vi "desacade.vi"(0 "Data not diff":dbl[][](array[numeric]), 2 "Capture Saccades":bool, 7 "desacc":T2={"Threshold 1 [Acc]"=0.0, "Threshold 2 [% of TH1]"=0, "tolerance"=2.0, "Search WD "=0.05757575757575758, " always use TH2"=TRUE, "SD for Outliers"=3.0303030303030303, "Max time [ms]"=50.0, "Min time [ms]"=1.0, "Velocity Threshold"=0.05757575757575758} {"Velocity Threshold" scale=50.0..400.0; "SD for Outliers" scale=0.0..5.0; "Search WD" scale=0.0..0.3; "tolerance" scale=0.0..100.0; "Threshold 2 [% of TH1]" scale=0.0..100.0; "Threshold 1 [Acc]" scale=1.0..40000.0}, 9 "Impulse Direction +ve?":bool, 11 "Sample Rate":dbl=500.0 format="%.2f", 12 "Impulse Positions":T1(array[cluster])=[{"Start"=-31, "End"=518, "Impulse Plane"=enum."Other", "Impulse Direction +ve?"=TRUE, "Time offset"=0, "Amplitude offset"=0.0}, {"Start"=369, "End"=913, "Impulse Plane"=enum."Other", "Impulse Direction +ve?"=TRUE, "Time offset"=0, "Amplitude offset"=0.0}, {"Start"=570, "End"=1018, "Impulse Plane"=enum."Other", "Impulse Direction +ve?"=FALSE, "Time offset"=0, "Amplitude offset"=0.0}, {"Start"=770, "End"=1311, "Impulse Plane"=enum."Other", "Impulse Direction +ve?"=TRUE, "Time offset"=0, "Amplitude offset"=0.0}, {"Start"=969, "End"=1417, "Impulse Plane"=enum."Other", "Impulse Direction +ve?"=FALSE, "Time offset"=0, "Amplitude offset"=0.0}, {"Start"=1170, "End"=1708, "Impulse Plane"=enum."Other", "Impulse Direction +ve?"=TRUE, "Time offset"=0, "Amplitude offset"=0.0}, {"Start"=1371, "End"=1819, "Impulse Plane"=enum."Other", "Impulse Direction +ve?"=FALSE, "Time offset"=0, "Amplitude offset"=0.0}, {"Start"=1570, "End"=2104, "Impulse Plane"=enum."Other", "Impulse Direction +ve?"=TRUE, "Time offset"=0, "Amplitude offset"=0.0}, {"Start"=1770, "End"=2218, "Impulse Plane"=enum."Other", "Impulse Direction +ve?"=FALSE, "Time offset"=0, "Amplitude offset"=0.0}, {"Start"=1971, "End"=2508, "Impulse Plane"=enum."Other", "Impulse Direction +ve?"=TRUE, "Time offset"=0, "Amplitude offset"=0.0}, {"Start"=2171, "End"=2619, "Impulse Plane"=enum."Other", "Impulse Direction +ve?"=FALSE, "Time offset"=0, "Amplitude offset"=0.0}, {"Start"=2370, "End"=2917, "Impulse Plane"=enum."Other", "Impulse Direction +ve?"=TRUE, "Time offset"=0, "Amplitude offset"=0.0}, {"Start"=2571, "End"=3019, "Impulse Plane"=enum."Other", "Impulse Direction +ve?"=FALSE, "Time offset"=0, "Amplitude offset"=0.0}, {"Start"=2771, "End"=3308, "Impulse Plane"=enum."Other", "Impulse Direction +ve?"=TRUE, "Time offset"=0, "Amplitude offset"=0.0}, {"Start"=2970, "End"=3418, "Impulse Plane"=enum."Other", "Impulse Direction +ve?"=FALSE, "Time offset"=0, "Amplitude offset"=0.0}, {"Start"=3172, "End"=3715, "Impulse Plane"=enum."Other", "Impulse Direction +ve?"=TRUE, "Time offset"=0, "Amplitude offset"=0.0}, {"Start"=3372, "End"=3820, "Impulse Plane"=enum."Other", "Impulse Direction +ve?"=FALSE, "Time offset"=0, "Amplitude offset"=0.0}, {"Start"=3572, "End"=4107, "Impulse Plane"=enum."Other", "Impulse Direction +ve?"=TRUE, "Time offset"=0, "Amplitude offset"=0.0}, {"Start"=3772, "End"=4220, "Impulse Plane"=enum."Other", "Impulse Direction +ve?"=FALSE, "Time offset"=0, "Amplitude offset"=0.0}, {"Start"=3972, "End"=4512, "Impulse Plane"=enum."Other", "Impulse Direction +ve?"=TRUE, "Time offset"=0, "Amplitude offset"=0.0}, {"Start"=4172, "End"=4620, "Impulse Plane"=enum."Other", "Impulse Direction +ve?"=FALSE, "Time offset"=0, "Amplitude offset"=0.0}, {"Start"=4373, "End"=4920, "Impulse Plane"=enum."Other", "Impulse Direction +ve?"=TRUE, "Time offset"=0, "Amplitude offset"=0.0}, {"Start"=4572, "End"=5020, "Impulse Plane"=enum."Other", "Impulse Direction +ve?"=FALSE, "Time offset"=0, "Amplitude offset"=0.0}, {"Start"=4773, "End"=5315, "Impulse Plane"=enum."Other", "Impulse Direction +ve?"=TRUE, "Time offset"=0, "Amplitude offset"=0.0}, {"Start"=4973, "End"=5421, "Impulse Plane"=enum."Other", "Impulse Direction +ve?"=FALSE, "Time offset"=0, "Amplitude offset"=0.0}, {"Start"=5173, "End"=5716, "Impulse Plane"=enum."Other", "Impulse Direction +ve?"=TRUE, "Time offset"=0, "Amplitude offset"=0.0}, {"Start"=5373, "End"=5821, "Impulse Plane"=enum."Other", "Impulse Direction +ve?"=FALSE, "Time offset"=0, "Amplitude offset"=0.0}, {"Start"=5573, "End"=6110, "Impulse Plane"=enum."Other", "Impulse Direction +ve?"=TRUE, "Time offset"=0, "Amplitude offset"=0.0}, {"Start"=5773, "End"=6221, "Impulse Plane"=enum."Other", "Impulse Direction +ve?"=FALSE, "Time offset"=0, "Amplitude offset"=0.0}, {"Start"=5972, "End"=6515, "Impulse Plane"=enum."Other", "Impulse Direction +ve?"=TRUE, "Time offset"=0, "Amplitude offset"=0.0}, {"Start"=6174, "End"=6622, "Impulse Plane"=enum."Other", "Impulse Direction +ve?"=FALSE, "Time offset"=0, "Amplitude offset"=0.0}, {"Start"=6373, "End"=6913, "Impulse Plane"=enum."Other", "Impulse Direction +ve?"=TRUE, "Time offset"=0, "Amplitude offset"=0.0}, {"Start"=6574, "End"=7022, "Impulse Plane"=enum."Other", "Impulse Direction +ve?"=FALSE, "Time offset"=0, "Amplitude offset"=0.0}, {"Start"=6774, "End"=7314, "Impulse Plane"=enum."Other", "Impulse Direction +ve?"=TRUE, "Time offset"=0, "Amplitude offset"=0.0}, {"Start"=6974, "End"=7422, "Impulse Plane"=enum."Other", "Impulse Direction +ve?"=FALSE, "Time offset"=0, "Amplitude offset"=0.0}, {"Start"=7175, "End"=7712, "Impulse Plane"=enum."Other", "Impulse Direction +ve?"=TRUE, "Time offset"=0, "Amplitude offset"=0.0}, {"Start"=7374, "End"=7822, "Impulse Plane"=enum."Other", "Impulse Direction +ve?"=FALSE, "Time offset"=0, "Amplitude offset"=0.0}, {"Start"=7574, "End"=8111, "Impulse Plane"=enum."Other", "Impulse Direction +ve?"=TRUE, "Time offset"=0, "Amplitude offset"=0.0}, {"Start"=7774, "End"=8222, "Impulse Plane"=enum."Other", "Impulse Direction +ve?"=FALSE, "Time offset"=0, "Amplitude offset"=0.0}, {"Start"=7974, "End"=8518, "Impulse Plane"=enum."Other", "Impulse Direction +ve?"=TRUE, "Time offset"=0, "Amplitude offset"=0.0}, {"Start"=8175, "End"=8623, "Impulse Plane"=enum."Other", "Impulse Direction +ve?"=FALSE, "Time offset"=0, "Amplitude offset"=0.0}, {"Start"=8375, "End"=8920, "Impulse Plane"=enum."Other", "Impulse Direction +ve?"=TRUE, "Time offset"=0, "Amplitude offset"=0.0}, {"Start"=8575, "End"=9023, "Impulse Plane"=enum."Other", "Impulse Direction +ve?"=FALSE, "Time offset"=0, "Amplitude offset"=0.0}, {"Start"=8776, "End"=9315, "Impulse Plane"=enum."Other", "Impulse Direction +ve?"=TRUE, "Time offset"=0, "Amplitude offset"=0.0}, {"Start"=8975, "End"=9423, "Impulse Plane"=enum."Other", "Impulse Direction +ve?"=FALSE, "Time offset"=0, "Amplitude offset"=0.0}, {"Start"=9176, "End"=9715, "Impulse Plane"=enum."Other", "Impulse Direction +ve?"=TRUE, "Time offset"=0, "Amplitude offset"=0.0}, {"Start"=9375, "End"=9823, "Impulse Plane"=enum."Other", "Impulse Direction +ve?"=FALSE, "Time offset"=0, "Amplitude offset"=0.0}, {"Start"=9575, "End"=10110, "Impulse Plane"=enum."Other", "Impulse Direction +ve?"=TRUE, "Time offset"=0, "Amplitude offset"=0.0}], 13 "Display Saccades":bool) -> (4 "Desaccaded":dbl[][](graph), 6 "Mean":dbl[](graph), 8 "STD":dbl[](array[numeric]) format="%.2f", 10 "Mean and STD":dbl[][](array[numeric]) format="%.2f", 14 "Impulse Positions 2":T1(array[cluster]), 15 "Mean (-inf)":dbl[](array[numeric]) format="%.2f")   [LabVIEW 2016]
uses:
  <vilib>/Analysis/3filter.llb/Savitzky-Golay Filter (DBL).vi
  <vilib>/Analysis/NI_AALPro.lvlib
  <vilib>/Analysis/NI_AALBase.lvlib
  stats/stats.lvlib
  nan operations/nan operations.lvlib
panel:
  out "Desaccaded 4":dbl[](graph)
  out "Desaccaded 3":dbl[][](graph)
  out "Desaccaded 2":dbl[](graph)
  out "Data Diff & Quadr - Unsmoothed":dbl[][](graph)
  out "Data DIff & Quadr - Smoothed":dbl[][](graph)
  out "Data not differentiated":dbl[][](graph)
  # "Data Input"
  # "Mean and Standard deviation"
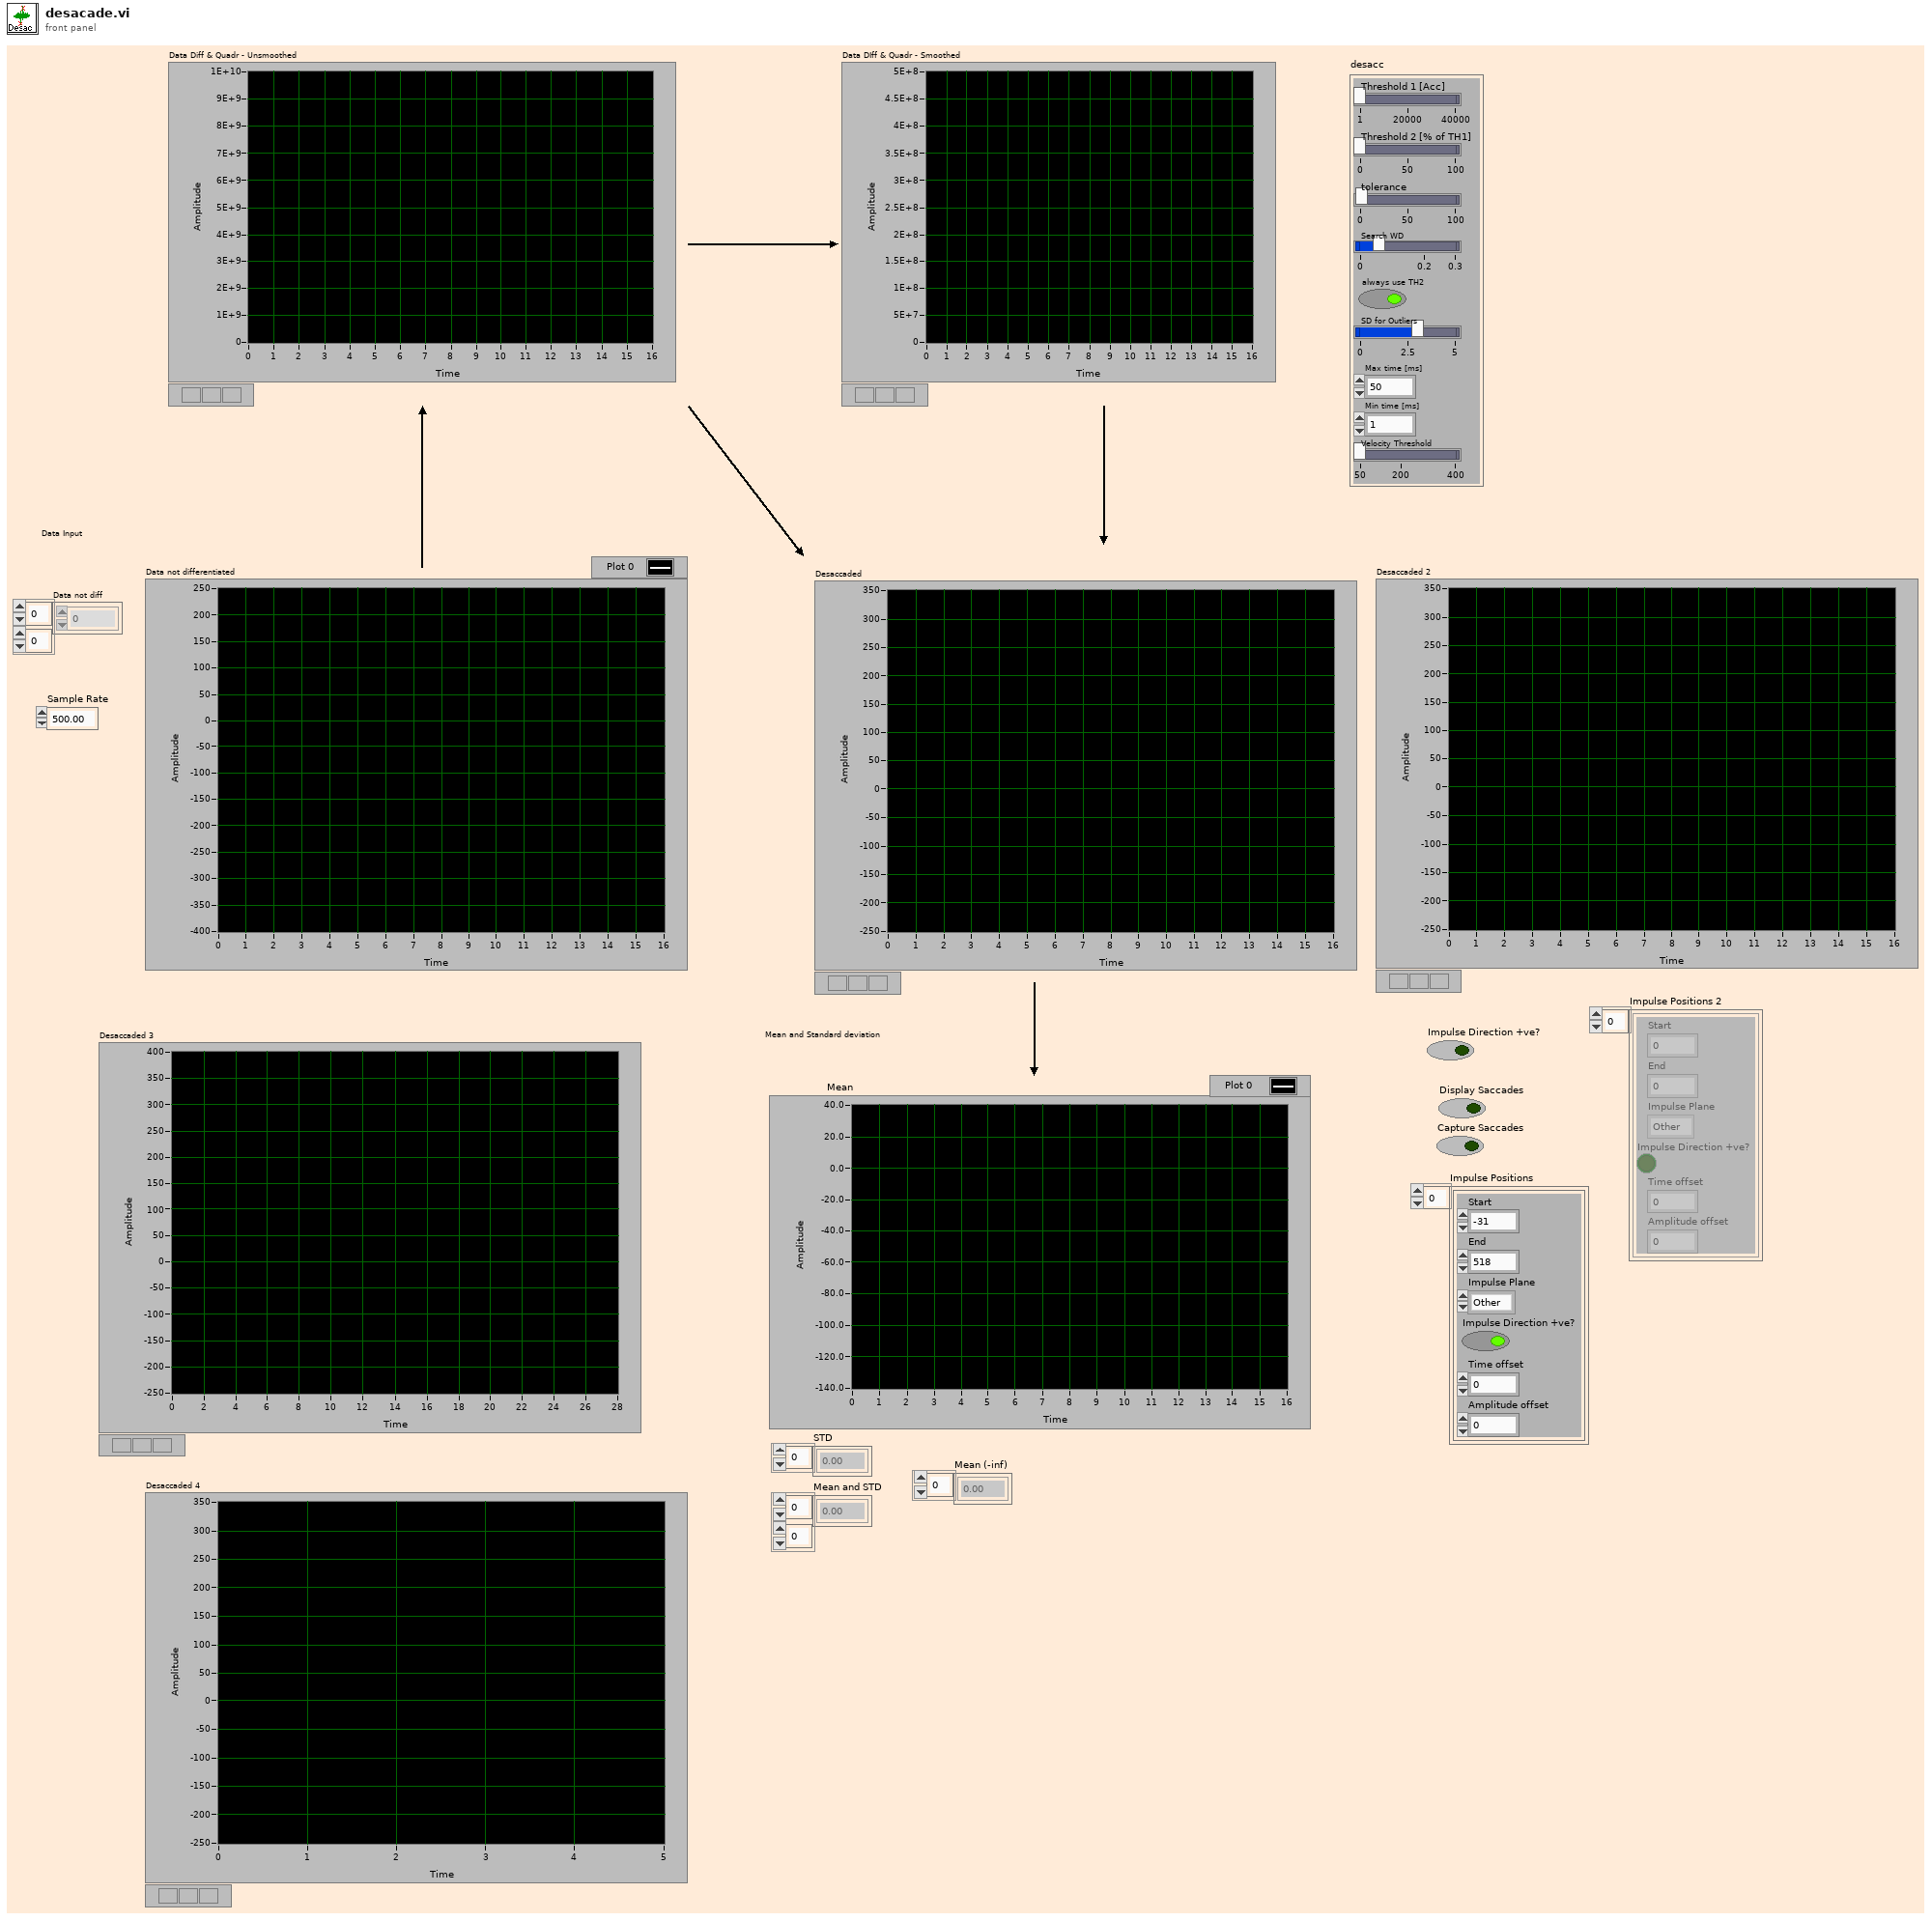
[diagram p1: front panel]
types:
  T1 = cluster{"Start":i32, "End":i32, "Impulse Plane":enum16{"Other", "Yaw", "Pitch", "Roll", "LARP", "RALP"}, "Impulse Direction +ve?":bool, "Time offset":i32, "Amplitude offset":dbl}[]
  T2 = cluster{"Threshold 1 [Acc]":dbl, "Threshold 2 [% of TH1]":i32, "tolerance":dbl, "Search WD ":dbl, " always use TH2":bool, "SD for Outliers":dbl, "Max time [ms]":dbl, "Min time [ms]":dbl, "Velocity Threshold":dbl}
  T3 = cluster{"Start":i32, "End":i32, "Impulse Plane":enum16{"Other", "Yaw", "Pitch", "Roll", "LARP", "RALP"}, "Impulse Direction +ve?":bool, "Time offset":i32, "Amplitude offset":dbl}
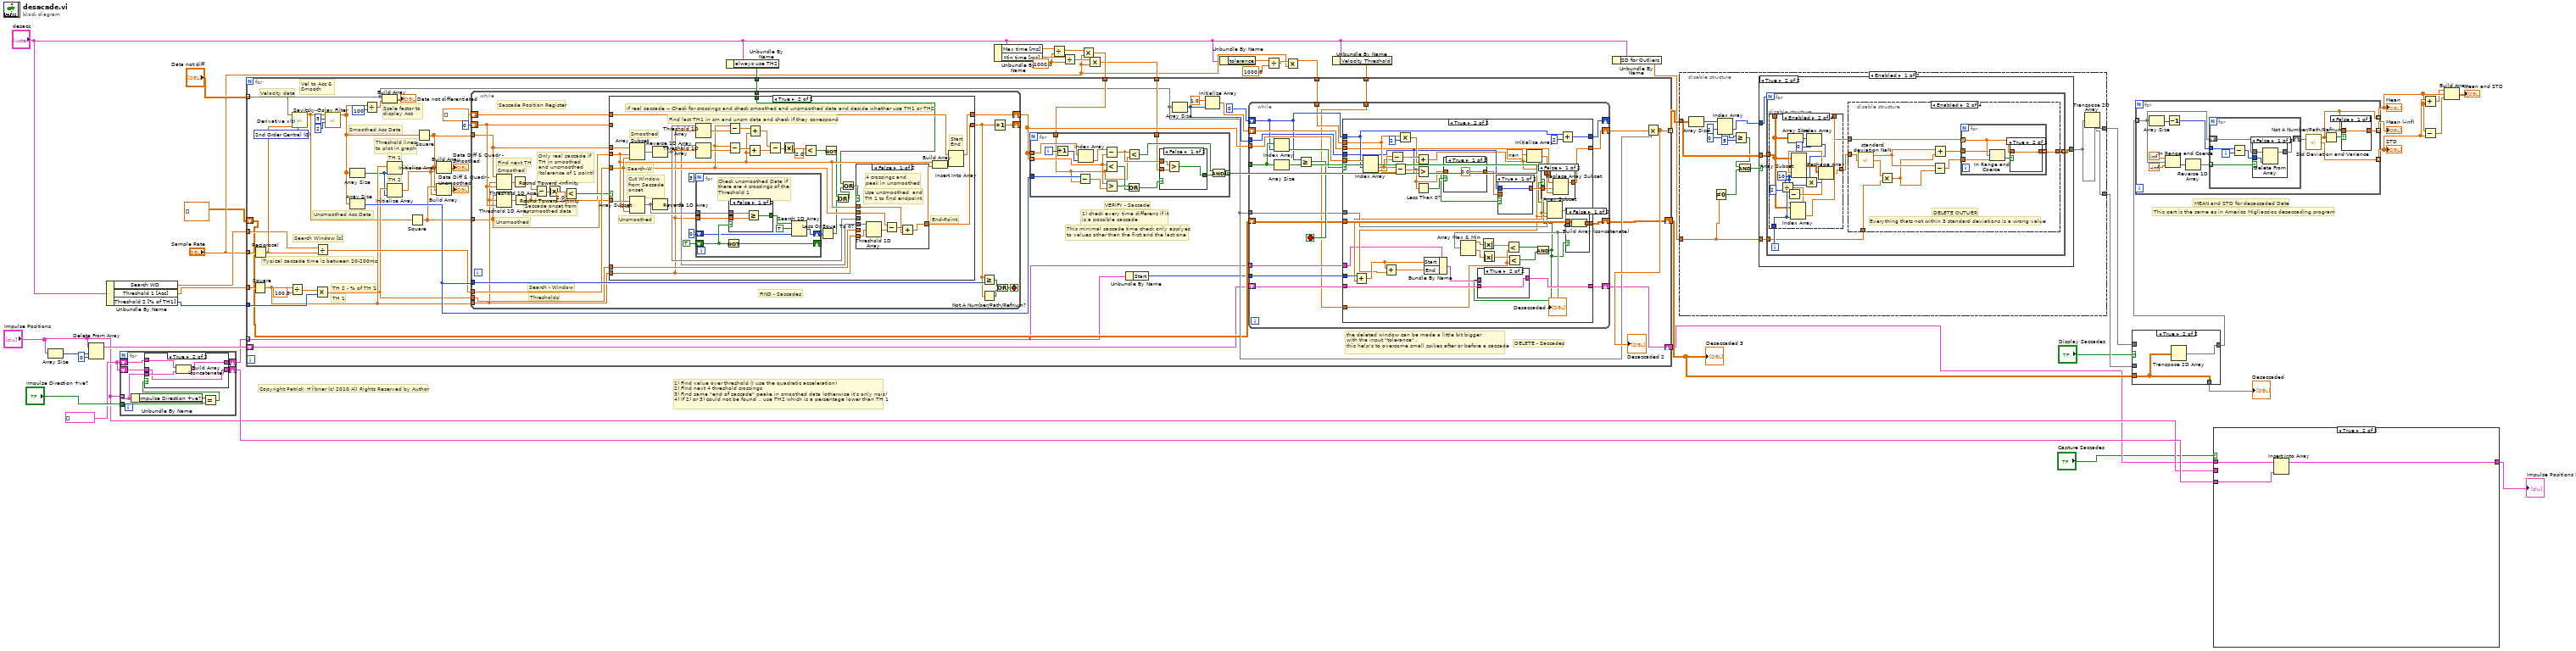
[diagram p0: block diagram]
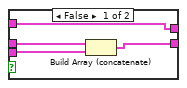
[diagram p3: hidden frame]
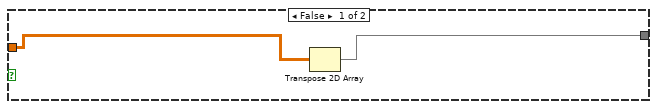
[diagram p5: hidden frame]
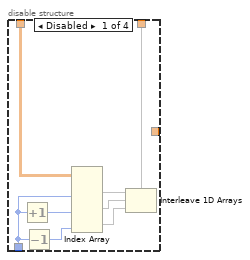
[diagram p6: hidden frame]
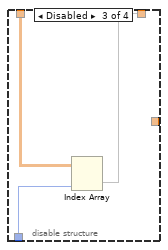
[diagram p7: hidden frame]
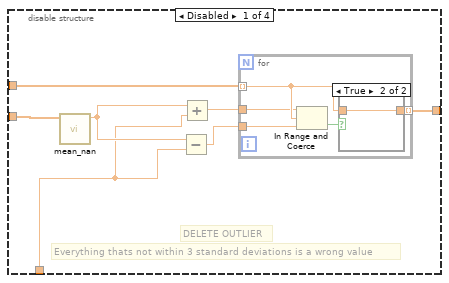
[diagram p9: hidden frame]
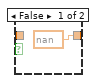
[diagram p10: hidden frame]
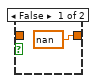
[diagram p11: hidden frame]
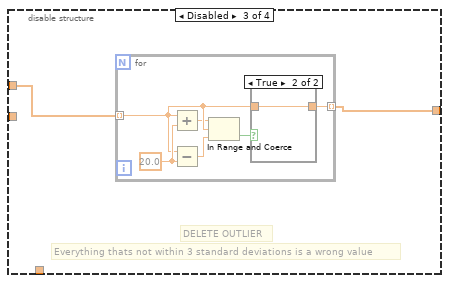
[diagram p12: hidden frame]
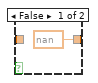
[diagram p13: hidden frame]
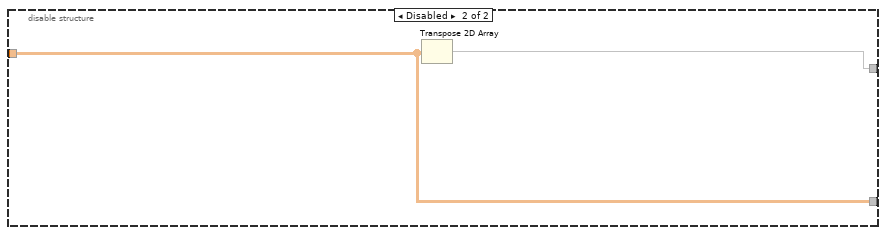
[diagram p15: hidden frame]
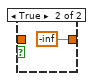
[diagram p17: hidden frame]
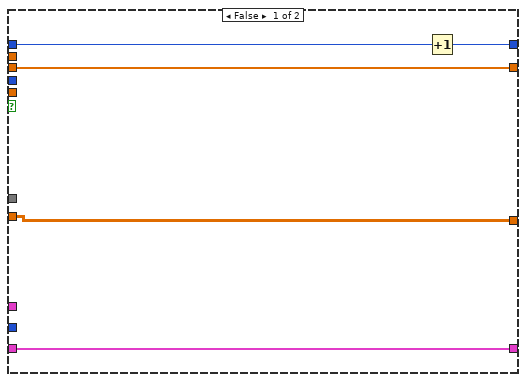
[diagram p18: hidden frame]
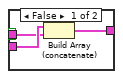
[diagram p20: hidden frame]
diagram:
  w8 = T1 []
  w30 = 1000.0 ("y")
  # "This part is the same as in Americo Migliaccios desaccading program"
  # "MEAN and STD for desaccaded Data"
  # "1) Find value over threshold (I use the quadratic acceleration)\n2) Find next 4 threshold crossings\n3) Find same \"end of saccade\" peake in smoothed data (otherwise it's only nois)\n4) If 2) or 3) could not be found .. use TH2 which is a persentage lower than TH 1"
  # "Copyright Patrick  HŸbner (c) 2010 All Rights Reserved by Author"
  n1 = Array Size(array="Impulse Positions") -> (size(s)=w11:i32)
  n2 = Delete From Array(array="Impulse Positions", length=w11, index=0) -> (array with subset deleted=w13:T1)  [unwired: 1 out]
  n3 = Unbundle By Name("desacc") -> ("Search WD"=w37:dbl, "Threshold 1 [Acc]"=w36:dbl, "Threshold 2 [% of TH1]"=w35:i32)
  n4 = for {
    tunnel: "Impulse Positions" -> [w48] mode=indexing
    tunnel: "Impulse Direction +ve?" -> [w52]
    shift-right: [w49] -> w9
    shift-left: w8 -> [w50]
    shift-right: [w46] -> w7
    shift-left: w8 -> [w47]
    n5 = Unbundle By Name(w48) -> ("Impulse Direction +ve?"=w53:bool)
    n6 = Equal?(x=w53, y=w52) -> (x = y?=w51:bool)
    n7 = case shown="True" w51 {
      tunnel: w48 -> [w56 w61]
      tunnel: w50 -> [w57 w60]
      tunnel: [w57 w59] -> w49
      tunnel: w47 -> [w55 w58]
      tunnel: [w54 w58] -> w46
      frame False {
        n8 = Build Array (concatenate)(w55, w56) -> (w54:T1)
      }
      frame True {
        n9 = Build Array (concatenate)(w60, w61) -> (w59:T1)
      }
    }
  }
  n10 = Unbundle By Name("desacc") -> ("always use TH2"=w34:bool)
  n11 = Unbundle By Name("desacc") -> ("Max time [ms]"=w32:dbl, "Min time [ms]"=w31:dbl)
  n12 = Divide(x=w32, y=w30) -> (x/y=w29:dbl)
  n13 = Divide(x=w31, y=w30) -> (x/y=w28:dbl)
  n14 = Multiply(x=w29, y="Sample Rate") -> (x*y=w27:dbl)
  n15 = Multiply(x=w28, y="Sample Rate") -> (x*y=w26:dbl)
  n16 = Unbundle By Name("desacc") -> ("tolerance"=w25:dbl)
  n17 = Divide(x=w25, y=1000.0) -> (x/y=w22:dbl)
  n18 = Multiply(x=w22, y="Sample Rate") -> (x*y=w23:dbl)
  n19 = Unbundle By Name("desacc") -> ("Velocity Threshold"=w1:dbl)
  n20 = for {
    tunnel: "Sample Rate" -> [w109]
    tunnel: w36 -> [w106]
    tunnel: "Data not diff" -> [w70] mode=indexing
    tunnel: [w76] -> w38 mode=indexing
    tunnel: w35 -> [w92]
    tunnel: w37 -> [w75]
    tunnel: w34 -> [w74]
    tunnel: w27 -> [w73]
    tunnel: w23 -> [w72]
    tunnel: w26 -> [w71]
    shift-right: [w69] -> w17
    shift-left: dbl[][] [] -> [w68]
    tunnel: w9 -> [w67] mode=indexing
    shift-right: [w64] -> w5
    shift-left: w13 -> [w65]
    tunnel: w1 -> [w63]
    w108 = u16 0 items=["2nd Order Central", "4th Order Central", "Forward", "Backward"] ("method")
    # "DELETE - Saccades"
    # "Scale factor to \ndisplay Acc"
    # "This minimal saccade time check only applyes \nto values other than the first and the last one"
    # "VERIFY - Saccade"
    # "Threshold lines \nto plot in graph"
    # "TH 2"
    # "TH 1"
    # "Vel to Acc &\nSmooth"
    # "Unsmoothed Acc Data"
    # "Smoothed Acc Data"
    # "Velocity data"
    # "Typical saccade time is between 20-200ms"
    # "Search Window [s]"
    # "TH 1"
    # "TH 2 - % of TH 1"
    # "the deleted window can be made a little bit bigger \nwith the input \"tolerance\" . \nthis help's to overcome small spikes after or before a saccade"
    # "1) check every time differenz if it \nis a possible saccade"
    n21 = Square(x=w106) -> (x^2=w88:dbl)
    n22 = Reciprocal(x=w109) -> (1/x=w79:dbl)
    n23 = Divide(x=w88, y=100.0) -> (x/y=w93:dbl)
    n24 = call <vilib>:"Derivative x(t).vi"("method"=w108, "dt"=w79, "X"=w70) -> ("dX/dt"=w62:dbl[])  [unwired: 7 in, 1 out]
    n25 = Multiply(x=w93, y=w92) -> (x*y=w87:dbl)
    n26 = Divide(x=w75, y=w79) -> (x/y=w89:dbl)
    n27 = call-poly <vilib>:"Savitzky-Golay Filter.vi"("polynomial order"=2, "side points"=5, "X"=w62) -> ("Filtered X"=w78:dbl[])  [unwired: 7 in, 1 out]
    n28 = Array Size(array=w78) -> (size(s)=w86:i32)
    n29 = Array Size(array=w78) -> (size(s)=w99:i32)
    n30 = Divide(x=w78, y=100 ("Numeric")) -> (x/y=w96:dbl[])
    n31 = Build Array(w70, w96) -> (→"Data not differentiated":dbl[][])
    n32 = Initialize Array(w88, w86) -> (w81:dbl[])
    n33 = Initialize Array(w87, w86) -> (w80:dbl[])
    n34 = Square(x=w62) -> (x^2=w83:dbl[])
    n35 = Square(x=w78) -> (x^2=w82:dbl[])
    n36 = Build Array(w82, w81, w80) -> (→"Data DIff & Quadr - Smoothed":dbl[][])
    n37 = Build Array(w83, w81, w80) -> (→"Data Diff & Quadr - Unsmoothed":dbl[][])
    n38 = while {
      tunnel: w82 -> [w217]
      shift-right: [w231] -> _
      shift-left: 0 -> [w220]
      shift-right: [w232] -> w101
      shift-left: dbl[] [] ("Filtered X") -> [w230]
      tunnel: w99 -> [w225]
      tunnel: w83 -> [w216]
      tunnel: w89 -> [w222]
      tunnel: w87 -> [w218]
      tunnel: w88 -> [w219]
      tunnel: w74 -> [w211]
      stop <- w224 stop-if-true
      # "FIND - Saccades"
      # "Saccade Position Register"
      # "Only real saccade if\nTH in smoothed\nand unsmoothed \n(tolerance of 1 point)"
      # "Unsmoothed"
      # "Smoothed"
      # "Saccade onset from\nunsmoothed data"
      # "Search - Window"
      # "Thresholds"
      # "Find next TH"
      n39 = Threshold 1D Array(1:w220, 2:w219, 3:w217) -> (0:w233:dbl)
      n40 = Threshold 1D Array(1:w220, 2:w219, 3:w216) -> (0:w229:dbl)
      n41 = Round Toward -Infinity(1:w233) -> (0:w215:dbl)
      n42 = Round Toward -Infinity(1:w229) -> (0:w214:dbl)
      n43 = Subtract(x=w215, y=w214) -> (x-y=w228:dbl)
      n44 = Absolute Value(x=w228) -> (abs(x)=w227:dbl)
      n45 = Less?(x=w227, y=2.0) -> (x < y?=w221:bool)
      n46 = case shown="True" w221 {
        tunnel: [w234 w268] -> w232
        tunnel: w230 -> [w234 w267]
        tunnel: w216 -> [_ w259]
        tunnel: w217 -> [_ w258]
        tunnel: w218 -> [_ w247]
        tunnel: [w235 w246] -> w223
        tunnel: w222 -> [_ w245]
        tunnel: w214 -> [_ w244]
        tunnel: w219 -> [_ w242]
        tunnel: w220 -> [w235 _]
        tunnel: w211 -> [_ w236]
        frame False {
          # "If no real saccade -- Do nothing"
        }
        frame True {
          # "End-Point"
          # "If real saccade -- Check for crossings and check smoothed and unsmoothed data and deside whether use TH1 or TH2"
          # "Find last TH1 in sm and unsm data and check if they correspond"
          # "Smoothed"
          # "Unsmoothed"
          # "Cut Window \nfrom Saccade\nonset"
          # "Search-W"
          # "Start\nEnd"
          n47 = Array Subset(array=w258, index=w244, length=w245) -> (w257:dbl[])
          n48 = Array Subset(array=w259, index=w244, length=w245) -> (w263:dbl[])
          n49 = Reverse 1D Array(array=w257) -> (reversed array=w248:dbl[])
          n50 = Reverse 1D Array(array=w263) -> (reversed array=w243:dbl[])
          n51 = Threshold 1D Array(2:w242, 3:w248) -> (0:w249:dbl)  [unwired: 1 in]
          n52 = Threshold 1D Array(2:w242, 3:w243) -> (0:w256:dbl)  [unwired: 1 in]
          n53 = for {
            N: 3 -> [_]
            tunnel: w263 -> [w290]
            shift-right: [w285] -> _
            shift-left: TRUE -> [w284]
            tunnel: w242 -> [w289]
            shift-right: [w286] -> w260
            shift-left: 0 ("index of element") -> [w283]
            # "Check unsmoothed Data if \nthere are 4 crossings of the \nThreshold 1"
            n54 = Not(x=w284) -> (.not. x?=w285:bool)
            n55 = case shown="False" w284 {
              tunnel: w290 -> [w293 w296]
              tunnel: w289 -> [w292 w295]
              tunnel: [w291 w294] -> w288
              frame False {
                n56 = Greater Or Equal?(x=w293, y=w292) -> (x >= y?=w291:bool[])
              }
              frame True {
                n57 = Less?(x=w296, y=w295) -> (x < y?=w294:bool[])
              }
            }
            n58 = Search 1D Array(1D array=w288, element=TRUE, start index (0)=w283) -> (index of element=w286:i32)
          }
          n59 = Subtract(x=w245, y=w249) -> (x-y=w255:dbl)
          n60 = Subtract(x=w245, y=w256) -> (x-y=w265:dbl)
          n61 = Add(x=w265, y=w244) -> (x+y=w250:dbl)
          n62 = Add(x=w255, y=w244) -> (x+y=w251:dbl)
          n63 = Subtract(x=w251, y=w250) -> (x-y=w254:dbl)
          n64 = Absolute Value(x=w254) -> (abs(x)=w253:dbl)
          n65 = Less?(x=w253, y=2.0) -> (x < y?=w241:bool)
          n66 = Less Or Equal To 0?(x=w260) -> (x <= 0?=w240:bool)
          n67 = Not(x=w241) -> (.not. x?=w239:bool)
          n68 = Or(x=w239, y=w240) -> (x .or. y?=w238:bool)
          n69 = Or(x=w236, y=w238) -> (x .or. y?=w237:bool)
          n70 = case shown="False" w237 {
            tunnel: w248 -> [_ w280]
            tunnel: w247 -> [_ w279]
            tunnel: [w273 w278] -> w246
            tunnel: w245 -> [w272 w277]
            tunnel: w244 -> [w271 w276]
            tunnel: w243 -> [w270 _]
            tunnel: w242 -> [w269 _]
            frame False {
              # "Use unsmoothed  and\nTH 1 to find endpoint"
              # "4 crossings and\npeak in unsmoothed"
              n71 = Threshold 1D Array(2:w269, 3:w270) -> (0:w274:dbl)  [unwired: 1 in]
              n72 = Subtract(x=w272, y=w274) -> (x-y=w275:dbl)
              n73 = Add(x=w275, y=w271) -> (x+y=w273:dbl)
            }
            frame True {
              # "Use smoothed data and\nTH 2 to find endpoint"
              # "not 4 crossings or \nno peak in unsmoothed"
              n74 = Threshold 1D Array(2:w279, 3:w280) -> (0:w281:dbl)  [unwired: 1 in]
              n75 = Subtract(x=w277, y=w281) -> (x-y=w282:dbl)
              n76 = Add(x=w282, y=w276) -> (x+y=w278:dbl)
            }
          }
          n77 = Build Array(w244, w246) -> (w266:dbl[])
          n78 = Insert Into Array(array=w267, new element=w266) -> (w268:dbl[])  [unwired: 1 in]
        }
      }
      n79 = Greater Or Equal?(x=w223, y=w225) -> (x >= y?=w213:bool)
      n80 = Not A Number/Path/Refnum?(number/path/refnum=w223) -> (NaN/Path/Refnum?=w212:bool)
      n81 = Increment(x=w223) -> (x+1=w231:dbl)
      n82 = Or(x=w213, y=w212) -> (x .or. y?=w224:bool)
    }
    n83 = for {
      tunnel: w101 -> [w195] mode=indexing
      tunnel: w101 -> [w206]
      tunnel: [w201] -> w104 mode=indexing
      tunnel: w99 -> [w193]
      tunnel: w73 -> [w192]
      tunnel: w71 -> [w191]
      i -> [w199]
      n84 = Increment(x=w199) -> (x+1=w205:i32)
      n85 = Subtract(x=w193, y=w192) -> (x-y=w194:dbl)
      n86 = Index Array(array=w206, index=w205) -> (element=w204:dbl)
      n87 = Subtract(x=w204, y=w195) -> (x-y=w200:dbl)
      n88 = Less?(x=w195, y=w192) -> (x < y?=w196:bool)
      n89 = Greater?(x=w195, y=w194) -> (0:w198:bool)
      n90 = Less?(x=w200, y=w192) -> (x < y?=w203:bool)
      n91 = Or(x=w198, y=w196) -> (x .or. y?=w197:bool)
      n92 = case shown="False" w197 {
        tunnel: w191 -> [w209 _]
        tunnel: [w208 TRUE] -> w202
        tunnel: w200 -> [w207 _]
        frame False {
          n93 = Greater?(x=w207, y=w209) -> (0:w208:bool)
        }
        frame True {
        }
      }
      n94 = And(x=w203, y=w202) -> (x .and. y?=w201:bool)
    }
    n95 = Unbundle By Name(w67) -> ("Start"=w66:i32)
    n96 = Array Size(array=w70) -> (size(s)=w98:i32)
    n97 = Initialize Array(1.0 ("element"), w98) -> (w102:dbl[])
    n98 = while {
      tunnel: w101 -> [w127]
      shift-right: [w125] -> w77
      shift-left: w102 -> [w126]
      shift-right: [w123] -> _
      shift-left: 0 -> [w120]
      tunnel: w104 -> [w124]
      tunnel: w98 -> [w119]
      tunnel: w72 -> [w118]
      shift-right: [w117] -> w69
      shift-left: w68 -> [w116]
      tunnel: w70 -> [w115]
      tunnel: w67 -> [w114]
      tunnel: w66 -> [w113]
      shift-right: [w111] -> w64
      shift-left: w65 -> [w112]
      tunnel: w63 -> [w110]
      stop <- w122 stop-if-true
      n99 = Index Array(array=w124, index=w120) -> (element=w128:bool)
      n100 = Array Size(array=w124) -> (size(s)=w121:i32)
      n101 = Greater Or Equal?(x=w120, y=w121) -> (x >= y?=w122:bool)
      n102 = case shown="True" w128 {
        tunnel: w127 -> [_ w173]
        tunnel: w126 -> [w133 w152]
        tunnel: [w133 w168] -> w125
        tunnel: w120 -> [w132 w166]
        tunnel: [w131 w167] -> w123
        tunnel: w118 -> [_ w161]
        tunnel: w119 -> [_ w156]
        tunnel: [w130 w155] -> w117
        tunnel: w116 -> [w130 w154]
        tunnel: w115 -> [_ w153]
        tunnel: w114 -> [_ w146]
        tunnel: w113 -> [_ w151]
        tunnel: w112 -> [w129 w145]
        tunnel: [w129 w143] -> w111
        tunnel: w110 -> [_ w134]
        frame False {
          n103 = Increment(x=w132) -> (x+1=w131:i32)
        }
        frame True {
          n104 = Index Array(array=w173, index #1=w166) -> (element #1=w162:dbl, element #2=w172:dbl)  [unwired: 1 in]
          n105 = Subtract(x=w172, y=w162) -> (x-y=w170:dbl)
          n106 = Subtract(x=w162, y=w161) -> (x-y=w159:dbl)
          n107 = Multiply(x=w161, y=2) -> (x*y=w163:dbl)
          n108 = Add(x=w170, y=w163) -> (x+y=w148:dbl)
          n109 = Greater?(x=w159, y=w156) -> (0:w158:bool)
          n110 = Less Than 0?(x=w159) -> (x < 0?=w160:bool)
          n111 = case shown="True" w160 {
            tunnel: w159 -> [_ w190]
            tunnel: [0.0 w190] -> w157
            frame True {
            }
            frame False {
            }
          }
          n112 = case shown="True" w158 {
            tunnel: w157 -> [_ w188]
            tunnel: [w187 w188] -> w150
            tunnel: w156 -> [w187 _]
            frame True {
            }
            frame False {
            }
          }
          n113 = Add(x=w151, y=w150) -> (x+y=w149:dbl)
          n114 = Add(x=w149, y=w148) -> (x+y=w147:dbl)
          n115 = Bundle By Name(cluster=w146, "Start"=w149, "End"=w147) -> (w144:T3)
          n116 = Initialize Array(nan, w148) -> (w169:dbl[])
          n117 = Array Subset(array=w153, index=w150, length=w148) -> (w136:dbl[])
          "Desaccaded 4" <- w136
          n118 = Array Max & Min(array=w136) -> (max value=w142:dbl, min value=w141:dbl)  [unwired: 2 out]
          n119 = Absolute Value(x=w142) -> (abs(x)=w140:dbl)
          n120 = Absolute Value(x=w141) -> (abs(x)=w139:dbl)
          n121 = Less?(x=w140, y=w134) -> (x < y?=w138:bool)
          n122 = Less?(x=w139, y=w134) -> (x < y?=w137:bool)
          n123 = And(x=w138, y=w137) -> (x .and. y?=w135:bool)
          n124 = case shown="True" w135 {
            tunnel: w145 -> [w180 w181]
            tunnel: w144 -> [w179 _]
            tunnel: [w178 w181] -> w143
            frame False {
              n125 = Build Array (concatenate)(w180, w179) -> (w178:T1)
            }
            frame True {
            }
          }
          n126 = case shown="False" w135 {
            tunnel: w169 -> [w185 _]
            tunnel: [w184 w186] -> w168
            tunnel: w152 -> [w183 w186]
            tunnel: w150 -> [w182 _]
            frame False {
              n127 = Replace Array Subset(array=w183, new element=w185, index=w182) -> (w184:dbl[])
            }
            frame True {
            }
          }
          n128 = Add(x=w166, y=2) -> (x+y=w167:i32)
          n129 = case shown="False" w135 {
            tunnel: [w176 w177] -> w155
            tunnel: w154 -> [w175 w177]
            tunnel: w136 -> [w174 _]
            frame False {
              n130 = Build Array (concatenate)(w175, w174) -> (w176:dbl[][])
            }
            frame True {
            }
          }
        }
      }
    }
    n131 = Multiply(x=w77, y=w70) -> (x*y=w76:dbl[])
    "Desaccaded 2" <- w76
  }
  "Desaccaded 3" <- w17
  n132 = Unbundle By Name("desacc") -> ("SD for Outliers"=w33:dbl)
  n133 = disable-structure shown="Enabled" {
    disable-tunnel: [w307 w386] -> w16
    disable-tunnel: [w306 w385] -> w19
    disable-tunnel: w38 -> [w305 w385]
    disable-tunnel: w33 -> [w297 _]
    frame Enabled {
      n134 = Array Size(array=w305) -> (size(s)=w309:i32[])
      n135 = Not Equal To 0?(x=w297) -> (x != 0?=w298:bool)
      n136 = Index Array(array=w309, index #1=1 ("index"), index #2=0 ("index")) -> (element #1=w304:i32, element #2=w302:i32)
      n137 = Greater Or Equal?(x=w302, y=5) -> (x >= y?=w299:bool)
      n138 = And(x=w299, y=w298) -> (x .and. y?=w300:bool)
      n139 = case shown="True" w300 {
        tunnel: [w310 w315] -> w307
        tunnel: w305 -> [w311 w314]
        tunnel: w304 -> [_ w313]
        tunnel: w297 -> [_ w312]
        frame False {
          n140 = Transpose 2D Array(2D array=w311) -> (transposed array=w310:dbl[][])
        }
        frame True {
          n141 = for {
            N: w313 -> [_]
            tunnel: w314 -> [w320]
            tunnel: [w321] -> w315 mode=indexing
            tunnel: w312 -> [w317]
            i -> [w318]
            n142 = disable-structure shown="Enabled" {
              disable-tunnel: w320 -> [w328 w334 w344 _]
              disable-tunnel: [w324 w341 w342 _] -> w319
              disable-tunnel: w318 -> [w322 w338 w343 _]
              disable-tunnel: [_ w336 _ _] -> w316
              frame Disabled {
                n143 = Increment(x=w322) -> (x+1=w327:i32)
                n144 = Decrement(x=w322) -> (x-1=w323:i32)
                n145 = Index Array(array=w328, index (col) #1=w322, index (col) #2=w327, index (col) #3=w323) -> (element #1=w324:dbl[], element #2=w326:dbl[], element #3=w325:dbl[])  [unwired: 3 in]
                n146 = Interleave 1D Arrays(w324, w326, w325) -> ()  [unwired: 1 out]
              }
              frame Enabled {
                w332 = 10 ("length")
                n147 = Divide(x=w332, y=2) -> (x/y=w337:dbl)
                n148 = Subtract(x=w338, y=w337) -> (x-y=w340:dbl)
                n149 = Array Size(array=w334) -> (size(s)=w331:i32[])
                n150 = Index Array(array=w334, index (col)=w338) -> (element=w341:dbl[])  [unwired: 1 in]
                n151 = Array Subset(array=w334, index (col)=w340, length (col)=w332) -> (w335:dbl[][])  [unwired: 2 in]
                n152 = Index Array(array=w331, index=0) -> (element=w330:i32)
                n153 = Multiply(x=w330, y=w332) -> (x*y=w329:i32)
                n154 = Reshape Array(w335, w329) -> (w336:dbl[])
              }
              frame Disabled {
                n155 = Index Array(array=w344, index (col)=w343) -> (element=w342:dbl[])  [unwired: 1 in]
              }
              frame Disabled {
              }
            }
            n156 = disable-structure shown="Enabled" {
              disable-tunnel: [w351 w367 w376 _] -> w321
              disable-tunnel: w316 -> [w350 w366 _ _]
              disable-tunnel: w319 -> [w349 w365 w375 _]
              disable-tunnel: w317 -> [w345 w360 _ _]
              frame Disabled {
                # "DELETE OUTLIER"
                # "Everything thats not within 3 standard deviations is a wrong value"
                n157 = call "mean_nan.vi"("Array"=w350) -> ("Mean"=w348:dbl)  [unwired: 10 in]
                n158 = Subtract(x=w348, y=w345) -> (x-y=w347:dbl)
                n159 = Add(x=w348, y=w345) -> (x+y=w346:dbl)
                n160 = for {
                  tunnel: [w355] -> w351 mode=indexing
                  tunnel: w349 -> [w354] mode=indexing
                  tunnel: w347 -> [w353]
                  tunnel: w346 -> [w352]
                  n161 = In Range and Coerce(upper limit=w352, x=w354, lower limit=w353) -> (In Range?=w356:bool)  [unwired: 1 out]
                  n162 = case shown="True" w356 {
                    tunnel: [nan w358] -> w355
                    tunnel: w354 -> [_ w358]
                    frame False {
                    }
                    frame True {
                    }
                  }
                }
              }
              frame Enabled {
                # "DELETE OUTLIER"
                # "Everything thats not within 3 standard deviations is a wrong value"
                n163 = call "standard deviation NaN.vi"("Array"=w366) -> ("standard deviation"=w361:dbl, "mean"=w364:dbl)  [unwired: 2 in, 1 out]
                n164 = Multiply(x=w361, y=w360) -> (x*y=w359:dbl)
                n165 = Subtract(x=w364, y=w359) -> (x-y=w363:dbl)
                n166 = Add(x=w364, y=w359) -> (x+y=w362:dbl)
                n167 = for {
                  tunnel: [w371] -> w367 mode=indexing
                  tunnel: w365 -> [w370] mode=indexing
                  tunnel: w363 -> [w369]
                  tunnel: w362 -> [w368]
                  n168 = In Range and Coerce(upper limit=w368, x=w370, lower limit=w369) -> (In Range?=w372:bool)  [unwired: 1 out]
                  n169 = case shown="True" w372 {
                    tunnel: [nan w374] -> w371
                    tunnel: w370 -> [_ w374]
                    frame False {
                    }
                    frame True {
                    }
                  }
                }
              }
              frame Disabled {
                # "DELETE OUTLIER"
                # "Everything thats not within 3 standard deviations is a wrong value"
                n170 = for {
                  tunnel: [w381] -> w376 mode=indexing
                  tunnel: w375 -> [w379] mode=indexing
                  w380 = 20.0 ("y")
                  n171 = Add(x=w379, y=w380) -> (x+y=w377:dbl)
                  n172 = Subtract(x=w379, y=w380) -> (x-y=w378:dbl)
                  n173 = In Range and Coerce(upper limit=w377, x=w379, lower limit=w378) -> (In Range?=w382:bool)  [unwired: 1 out]
                  n174 = case shown="True" w382 {
                    tunnel: [nan w384] -> w381
                    tunnel: w379 -> [_ w384]
                    frame False {
                    }
                    frame True {
                    }
                  }
                }
              }
              frame Disabled {
              }
            }
          }
        }
      }
      n175 = Transpose 2D Array(2D array=w307) -> (transposed array=w306:dbl[][])
    }
    frame Disabled {
      n176 = Transpose 2D Array(2D array=w385) -> (transposed array=w386:dbl[][])
    }
  }
  n177 = case shown="True" "Display Saccades" {
    tunnel: w19 -> [w388 _]
    tunnel: [w388 w389] -> w18
    tunnel: w17 -> [_ w389]
    tunnel: [w387 w390] -> w15
    tunnel: w16 -> [w387 _]
    frame False {
    }
    frame True {
      n178 = Transpose 2D Array(2D array=w389) -> (transposed array=w390:dbl[][])
    }
  }
  "Desaccaded" <- w18
  n179 = for {
    tunnel: w15 -> [w393] mode=indexing
    tunnel: [w399] -> w43 mode=indexing
    tunnel: [w402] -> w44 mode=indexing
    tunnel: [w400] -> w39 mode=indexing
    n180 = Array Size(array=w393) -> (size(s)=w392:i32)
    n181 = In Range and Coerce(upper limit=inf, x=w393, lower limit=-inf) -> (In Range?=w395:bool[])  [unwired: 1 out]
    n182 = Decrement(x=w392) -> (x-1=w391:i32)
    n183 = Reverse 1D Array(array=w395) -> (reversed array=w394:bool[])
    n184 = for {
      tunnel: w394 -> [w408] mode=indexing
      shift-right: [w406] -> w398
      shift-left: w393 -> [w407]
      tunnel: w391 -> [w405]
      i -> [w404]
      n185 = Subtract(x=w405, y=w404) -> (x-y=w403:i32)
      n186 = case shown="False" w408 {
        tunnel: w407 -> [w411 w412]
        tunnel: [w409 w412] -> w406
        tunnel: w403 -> [w410 _]
        frame False {
          n187 = Delete From Array(array=w411, index=w410) -> (array with subset deleted=w409:dbl[])  [unwired: 1 in, 1 out]
        }
        frame True {
        }
      }
    }
    n188 = call "Std Deviation and Variance.vi"("X"=w398) -> ("mean"=w399:dbl, "standard deviation"=w402:dbl)  [unwired: 1 in, 1 out]
    n189 = Not A Number/Path/Refnum?(number/path/refnum=w399) -> (NaN/Path/Refnum?=w401:bool)
    n190 = case shown="False" w401 {
      tunnel: [w413 -inf] -> w400
      tunnel: w399 -> [w413 _]
      frame False {
      }
      frame True {
      }
    }
  }
  "Mean" <- w43
  "STD" <- w44
  "Mean (-inf)" <- w39
  n191 = case shown="True" "Capture Saccades" {
    tunnel: w7 -> [_ w417]
    tunnel: "Impulse Positions" -> [w415 _]
    tunnel: w5 -> [_ w418]
    tunnel: [w415 w416] -> w4
    frame False {
    }
    frame True {
      n192 = Insert Into Array(array=w418, new element=w417) -> (w416:T1)  [unwired: 1 in]
    }
  }
  "Impulse Positions 2" <- w4
  n193 = Add(x=w44, y=w43) -> (x+y=w42:dbl[])
  n194 = Subtract(x=w43, y=w44) -> (x-y=w41:dbl[])
  n195 = Build Array(w42, w43, w41) -> (→"Mean and STD":dbl[][])
